vi "NiFPGA Read FIFO.vi"   [LabVIEW 2010, in "FPGA Interface Wrapper.lvlib"]
doc: "Reads data from a FIFO"
uses:
  <userlib>/_FPGA Interface Advanced Tools/FPGA Interface Wrapper/FPGA Interface Wrapper.lvlib
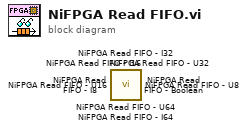
[diagram p0: block diagram]
diagram:
  n1 = call <userlib>:"NiFPGA Read FIFO - U64.vi"() -> ()  [unwired: 8 in, 4 out]
  n2 = call <userlib>:"NiFPGA Read FIFO - U32.vi"() -> ()  [unwired: 8 in, 4 out]
  n3 = call <userlib>:"NiFPGA Read FIFO - U16.vi"() -> ()  [unwired: 8 in, 4 out]
  n4 = call <userlib>:"NiFPGA Read FIFO - U8.vi"() -> ()  [unwired: 8 in, 4 out]
  n5 = call <userlib>:"NiFPGA Read FIFO - I64.vi"() -> ()  [unwired: 8 in, 4 out]
  n6 = call <userlib>:"NiFPGA Read FIFO - I32.vi"() -> ()  [unwired: 8 in, 4 out]
  n7 = call <userlib>:"NiFPGA Read FIFO - I16.vi"() -> ()  [unwired: 8 in, 4 out]
  n8 = call <userlib>:"NiFPGA Read FIFO - I8.vi"() -> ()  [unwired: 8 in, 4 out]
  n9 = call <userlib>:"NiFPGA Read FIFO - Boolean.vi"() -> ()  [unwired: 8 in, 4 out]
